vi "Swerve Oper.vi"   [LabVIEW 2016]
uses:
  Robot Global Data.vi
types:
  T1 = typedef "WPI_DriverStationRobotMode2.ctl" = enum16{"Autonomous Disabled", "Autonomous Enabled", "Teleop Disabled", "Teleop Enabled", "Disconnected", "Finish", "Test Disabled", "Test Enabled", "Emergency Stopped"}
  T2 = enum16{"X-axis", "Y-axis", "LTrigger", "RTrigger", "R-Xaxis", "R-Yaxis"}
  T3 = enum16{"A-but", "B-but", "Xbut", "Y-but", "L-but", "R_but"}
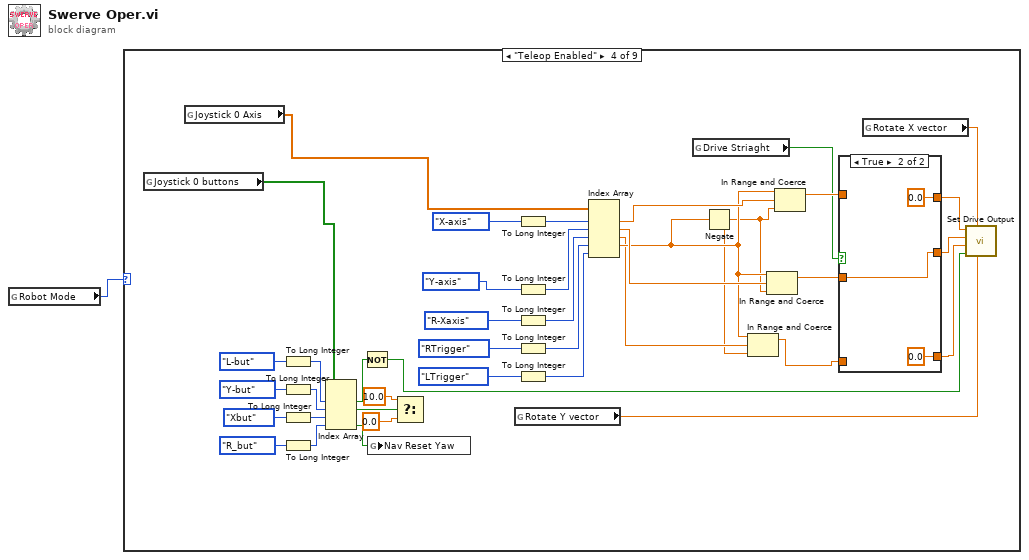
[diagram p0: block diagram]
diagram:
  n1 = global read "Robot Global Data.vi" "Robot Mode"() -> (w1:T1)
  n2 = case shown="\"Teleop Enabled\"" w1 {
    frame "Autonomous Disabled", Default {
    }
    frame "Autonomous Enabled" {
    }
    frame "Teleop Disabled" {
    }
    frame "Teleop Enabled" {
      n3 = global read "Robot Global Data.vi" "Joystick 0 buttons"() -> (w10:bool[])
      n4 = global read "Robot Global Data.vi" "Joystick 0 Axis"() -> (w11:dbl[])
      n5 = To Long Integer(number=T3."L-but") -> (32bit integer=w37:i32)
      n6 = To Long Integer(number=T3."Y-but") -> (32bit integer=w36:i32)
      n7 = To Long Integer(number=T3."Xbut") -> (32bit integer=w35:i32)
      n8 = To Long Integer(number=T3."R_but") -> (32bit integer=w34:i32)
      n9 = Index Array(array=w10, index #1=w37, index #2=w36, index #3=w35, index #4=w34) -> (element #1=w29:bool, element #2=w33:bool, element #4=w30:bool)  [unwired: 1 out]
      n10 = Not(x=w29) -> (.not. x?=w13:bool)
      n11 = global write "Robot Global Data.vi" "Nav Reset Yaw"(w30) -> ()
      n12 = Select(t=10.0, s=w33, f=0.0) -> ()  [unwired: 1 out]
      n13 = global read "Robot Global Data.vi" "Rotate Y vector"() -> (w14:dbl)
      n14 = To Long Integer(number=T2."X-axis") -> (32bit integer=w26:i32)
      n15 = To Long Integer(number=T2."Y-axis") -> (32bit integer=w25:i32)
      n16 = To Long Integer(number=T2."R-Xaxis") -> (32bit integer=w24:i32)
      n17 = To Long Integer(number=T2."RTrigger") -> (32bit integer=w22:i32)
      n18 = To Long Integer(number=T2."LTrigger") -> (32bit integer=w20:i32)
      n19 = Index Array(array=w11, index #1=w26, index #2=w25, index #3=w24, index #4=w22, index #5=w20) -> (element #1=w19:dbl, element #2=w18:dbl, element #3=w16:dbl, element #4=w17:dbl)  [unwired: 1 out]
      n20 = global read "Robot Global Data.vi" "Drive Striaght"() -> (w2:bool)
      n21 = Negate(x=w17) -> (-x=w9:dbl)
      n22 = In Range and Coerce(upper limit=w17, x=w16, lower limit=w9) -> (coerced(x)=w8:dbl)  [unwired: 1 out]
      n23 = In Range and Coerce(upper limit=w17, x=w18, lower limit=w9) -> (coerced(x)=w6:dbl)  [unwired: 1 out]
      n24 = In Range and Coerce(upper limit=w17, x=w19, lower limit=w9) -> (coerced(x)=w5:dbl)  [unwired: 1 out]
      n25 = case shown="True" w2 {
        tunnel: w8 -> [w42 _]
        tunnel: [w42 0.0 ("Numeric")] -> w7
        tunnel: w6 -> [w43 w45]
        tunnel: [w43 w45] -> w3
        tunnel: w5 -> [w44 _]
        tunnel: [w44 0.0 ("Numeric")] -> w4
        frame False {
        }
        frame True {
        }
      }
      n26 = global read "Robot Global Data.vi" "Rotate X vector"() -> (w12:dbl)
      n27 = call "Set Drive Output.vi"("Rot. Point Y"=w14, "Rot. Point X"=w12, "Field Concentric"=w13, "Z"=w7, "Y"=w3, "X"=w4) -> ()  [unwired: 6 in]
    }
    frame "Disconnected" {
    }
    frame "Finish" {
    }
    frame "Test Disabled" {
    }
    frame "Test Enabled" {
    }
    frame "Emergency Stopped" {
    }
  }
